vi "N_max_forsed_bit32.vi"(3 "IN":u32 format="%b") -> (1 "N":u32 format="%b")   [LabVIEW 2019]
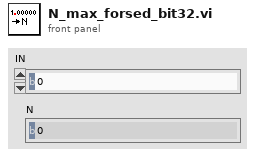
[diagram p1: front panel]
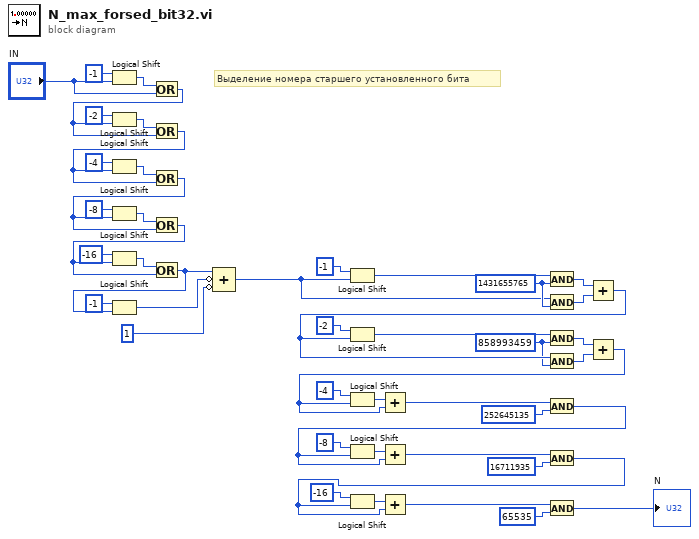
[diagram p0: block diagram]
diagram:
  w7 = u32 858993459 ("y")
  w4 = u32 1431655765 ("y")
  # "Выделение номера старшего установленного бита"
  n1 = Logical Shift(y=i16 -1, x="IN") -> (x << y=w40:u32)
  n2 = Or(x=w40, y="IN") -> (x .or. y?=w39:u32)
  n3 = Logical Shift(y=i16 -2, x=w39) -> (x << y=w47:u32)
  n4 = Or(x=w47, y=w39) -> (x .or. y?=w38:u32)
  n5 = Logical Shift(y=i16 -4, x=w38) -> (x << y=w44:u32)
  n6 = Or(x=w44, y=w38) -> (x .or. y?=w37:u32)
  n7 = Logical Shift(y=i16 -8, x=w37) -> (x << y=w43:u32)
  n8 = Or(x=w43, y=w37) -> (x .or. y?=w32:u32)
  n9 = Logical Shift(y=i16 -16, x=w32) -> (x << y=w33:u32)
  n10 = Or(x=w33, y=w32) -> (x .or. y?=w30:u32)
  n11 = Logical Shift(y=i16 -1, x=w30) -> (x << y=w36:u32)
  n12 = Compound Arithmetic op=ADD(w30, invert w36, invert u32 1 ("value")) -> (w3:u32)
  n13 = Logical Shift(y=i16 -1, x=w3) -> (x << y=w10:u32)
  n14 = And(x=w10, y=w4) -> (x .and. y?=w5:u32)
  n15 = And(x=w3, y=w4) -> (x .and. y?=w6:u32)
  n16 = Add(x=w5, y=w6) -> (x+y=w14:u32)
  n17 = Logical Shift(y=i16 -2, x=w14) -> (x << y=w13:u32)
  n18 = And(x=w13, y=w7) -> (x .and. y?=w8:u32)
  n19 = And(x=w14, y=w7) -> (x .and. y?=w9:u32)
  n20 = Add(x=w8, y=w9) -> (x+y=w17:u32)
  n21 = Logical Shift(y=i16 -4, x=w17) -> (x << y=w16:u32)
  n22 = Add(x=w16, y=w17) -> (x+y=w18:u32)
  n23 = And(x=w18, y=u32 252645135) -> (x .and. y?=w27:u32)
  n24 = Logical Shift(y=i16 -8, x=w27) -> (x << y=w22:u32)
  n25 = Add(x=w22, y=w27) -> (x+y=w21:u32)
  n26 = And(x=w21, y=u32 16711935) -> (x .and. y?=w28:u32)
  n27 = Logical Shift(y=i16 -16, x=w28) -> (x << y=w24:u32)
  n28 = Add(x=w24, y=w28) -> (x+y=w25:u32)
  n29 = And(x=w25, y=u32 65535) -> (x .and. y?=→"N":u32)
